vi "Xeryon serial data buffer.vi"(0 "Mode":T5(ring), 1 "Stage types in":string[][](array[string]), 2 "Position in":dbl, 5 "Drive letters in":string[](array[string]), 7 "Within tol in":bool, 9 "Parameters in":T2[](array[typedef]), 11 "Values in":i32[](array[numeric]), 12 "Select drive letter":string, 14 "Select parameter":T2) -> (3 "Stage data":T4(array[cluster]), 4 "Position out":dbl, 6 "Statusbits out":T1, 8 "Stage letters":string[](array[string]), 10 "Stage data":T3, 13 "Within tol out":bool, 15 "single value out":i32)   [LabVIEW 2014]
uses:
  Serial parameters.ctl
  Axis driver/Xeryon status bits.ctl
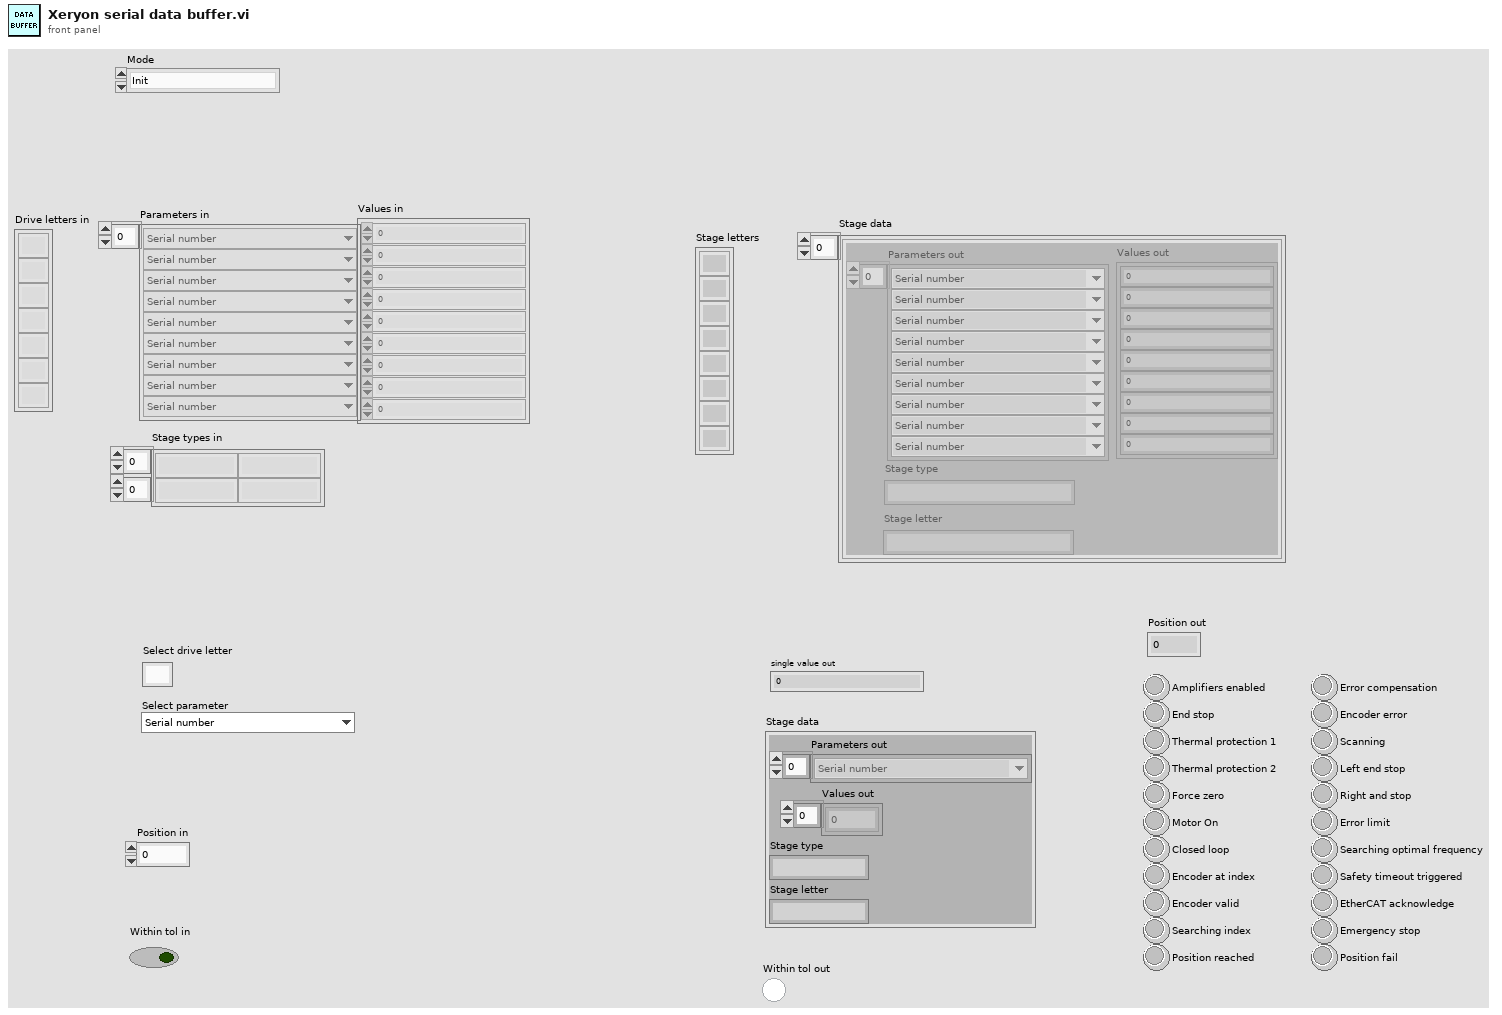
[diagram p1: front panel]
types:
  T1 = typedef "Xeryon status bits.ctl" = cluster{"Amplifiers enabled":bool, "End stop":bool, "Thermal protection 1":bool, "Thermal protection 2":bool, "Force zero":bool, "Motor On":bool, "Closed loop":bool, "Encoder at index":bool, "Encoder valid":bool, "Searching index":bool, "Position reached":bool, "Error compensation":bool, "Encoder error":bool, "Scanning":bool, "Left end stop":bool, "Right and stop":bool, "Error limit":bool, "Searching optimal frequency":bool, "Safety timeout triggered":bool, "EtherCAT acknowledge":bool, "Emergency stop":bool, "Position fail":bool}
  T2 = typedef "Serial parameters.ctl" = enum16{"Serial number", "Software number", "Type of stage", "Status", "Frequency", "Encoder position", "Desired position", "Info", "Phase correction", "Timestamp", "Proportional control factor", "Sync", "XRT1", "XRT3", "XRTA", "XLS1", "XLS3", "XLA1", "XLA3"}
  T3 = cluster{"Parameters out":T2[], "Values out":i32[], "Stage type":string, "Stage letter":string}
  T4 = cluster{"Parameters out":T2[], "Values out":i32[], "Stage type":string, "Stage letter":string}[]
  T5 = enum16{"Init", "Set stage data", "Update position", "Get"}
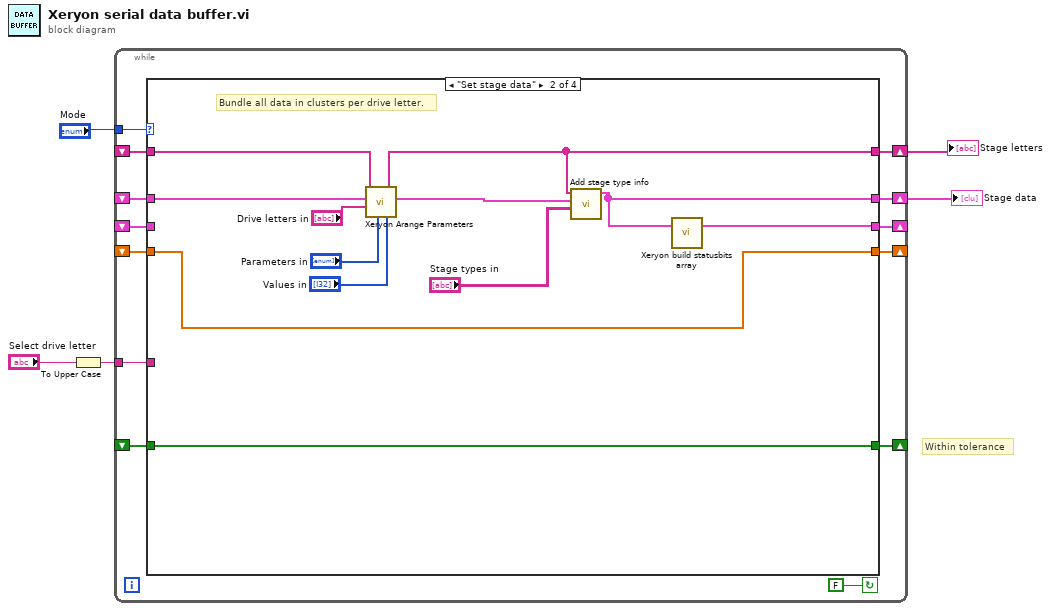
[diagram p0: block diagram]
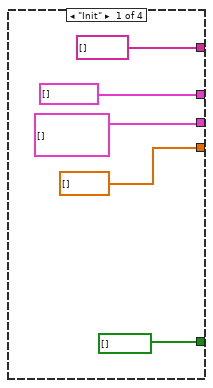
[diagram p2: hidden frame]
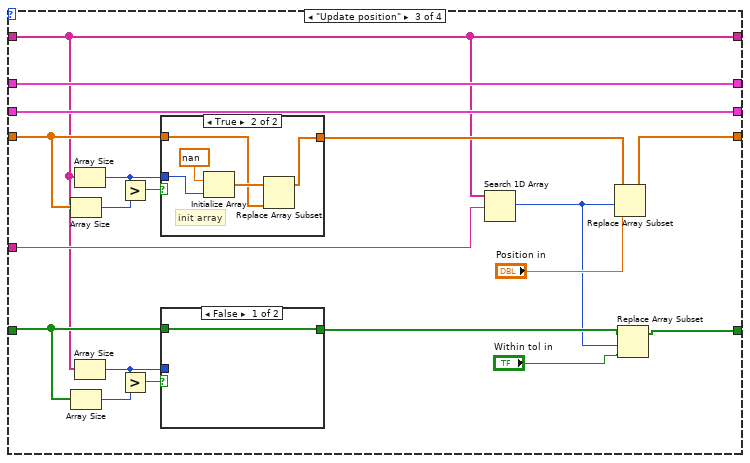
[diagram p3: hidden frame]
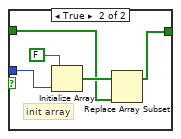
[diagram p4: hidden frame]
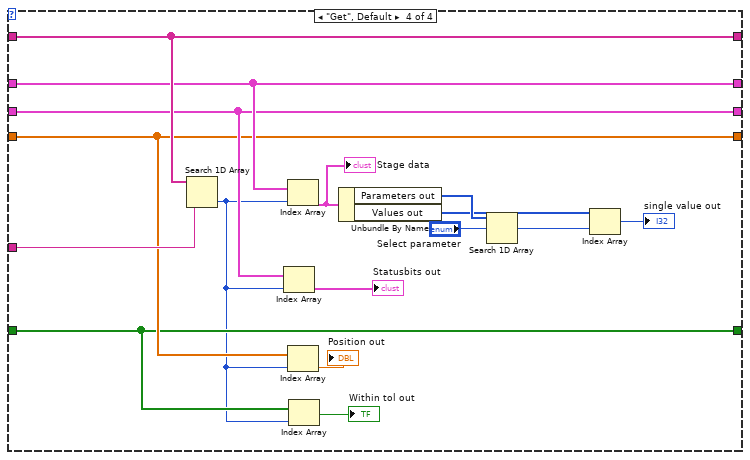
[diagram p6: hidden frame]
diagram:
  # "Within tolerance"
  n1 = To Upper Case(1:"Select drive letter") -> (0:w1:string)
  n2 = while {
    tunnel: "Mode" -> [w18]
    shift-right: [w14] -> w3
    shift-left: _ -> [w16]
    shift-right: [w13] -> w4
    shift-left: _ -> [w15]
    shift-right: [w12] -> _
    shift-left: _ -> [w11]
    tunnel: w1 -> [w10]
    shift-right: [w9] -> _
    shift-left: _ -> [w8]
    shift-right: [w7] -> _
    shift-left: _ -> [w6]
    stop <- FALSE continue-if-true
    n3 = case shown="\"Set stage data\"" w18 {
      tunnel: w16 -> [_ w35 w40 w81]
      tunnel: w15 -> [_ w33 w54 w80]
      tunnel: [string[] [] w28 w40 w81] -> w14
      tunnel: [T4 [] w27 w54 w80] -> w13
      tunnel: [T1[] [] w26 w53 w74] -> w12
      tunnel: w11 -> [_ _ w53 w74]
      tunnel: w10 -> [_ _ w52 w72]
      tunnel: [dbl[] [] w25 w51 w71] -> w9
      tunnel: w8 -> [_ w25 w47 w71]
      tunnel: [bool[] [] w24 w38 w69] -> w7
      tunnel: w6 -> [_ w24 w41 w69]
      frame "Init" {
      }
      frame "Set stage data" {
        # "Bundle all data in clusters per drive letter."
        n4 = call "Xeryon Arange Parameters.vi"("Parameters in"="Parameters in", "Values in"="Values in", "New drive letters"="Drive letters in", "Data in"=w33, "Known drive letters"=w35) -> ("Data out"=w30:T4, "Drive letters out"=w28:string[])  [unwired: 5 in]
        n5 = call "Add stage type info.vi"("Stage types in"="Stage types in", "Data in"=w30, "Drive letters in"=w28) -> ("Array out"=w27:T4)  [unwired: 8 in]
        n6 = call "Xeryon build statusbits array.vi"("Array in"=w27) -> ("Array"=w26:T1[])  [unwired: 2 in]
      }
      frame "Update position" {
        n7 = Array Size(array=w47) -> (size(s)=w49:i32)
        n8 = Array Size(array=w41) -> (size(s)=w42:i32)
        n9 = Array Size(array=w40) -> (size(s)=w46:i32)
        n10 = Array Size(array=w40) -> (size(s)=w44:i32)
        n11 = Greater?(x=w46, y=w49) -> (0:w48:bool)
        n12 = Greater?(x=w44, y=w42) -> (0:w43:bool)
        n13 = case shown="True" w48 {
          tunnel: w47 -> [w61 w63]
          tunnel: w46 -> [_ w65]
          tunnel: [w61 w62] -> w45
          frame False {
          }
          frame True {
            # "init array"
            n14 = Initialize Array(nan, w65) -> (w64:dbl[])
            n15 = Replace Array Subset(array=w64, new element=w63) -> (w62:dbl[])  [unwired: 1 in]
          }
        }
        n16 = case shown="False" w43 {
          tunnel: w41 -> [w55 w58]
          tunnel: w44 -> [_ w60]
          tunnel: [w55 w57] -> w39
          frame False {
          }
          frame True {
            # "init array"
            n17 = Initialize Array(FALSE, w60) -> (w59:bool[])
            n18 = Replace Array Subset(array=w59, new element=w58) -> (w57:bool[])  [unwired: 1 in]
          }
        }
        n19 = Search 1D Array(1D array=w40, element=w52) -> (index of element=w36:i32)  [unwired: 1 in]
        n20 = Replace Array Subset(array=w45, new element="Position in", index=w36) -> (w51:dbl[])
        n21 = Replace Array Subset(array=w39, new element="Within tol in", index=w36) -> (w38:bool[])
      }
      frame "Get", Default {
        n22 = Search 1D Array(1D array=w81, element=w72) -> (index of element=w68:i32)  [unwired: 1 in]
        n23 = Index Array(array=w74, index=w68) -> (element=→"Statusbits out":T1)
        n24 = Index Array(array=w80, index=w68) -> (element=w79:T3)
        "Stage data" <- w79
        n25 = Index Array(array=w71, index=w68) -> (element=→"Position out":dbl)
        n26 = Index Array(array=w69, index=w68) -> (element=→"Within tol out":bool)
        n27 = Unbundle By Name(w79) -> ("Parameters out"=w78:T2[], "Values out"=w75:i32[])
        n28 = Search 1D Array(1D array=w78, element="Select parameter") -> (index of element=w82:i32)  [unwired: 1 in]
        n29 = Index Array(array=w75, index=w82) -> (element=→"single value out":i32)
      }
    }
  }
  "Stage letters" <- w3
  "Stage data" <- w4
